vi "PCO_GetCOCRuntime.vi"(8 "error in (no error)":errorcluster {"code" format="%x"}, 11 "ph":u64) -> (0 "error out":errorcluster {"code" format="%x"}, 1 "dwTime_s":u32, 2 "ErrorMessage":i32 format="%x", 3 "ph out":u64, 5 "dwTime_ns":u32)   [LabVIEW 2020, in "SDK.lvlib" / "TimingControl.lvlib"]
doc: "<b>Description:</b>\nThis function can be used to calculate the current frame rate of the camera.\nThe returned values describe exactly how much time is required to take a single image. The resulting time is calculated inside the camera and depends on the settings of the timing and sensor parameters. To cover the full range of possible times it is splitted in two parts. Parameter dwTime_s gives the number of seconds and dwTime_ns gives the number of nano seconds in the range from 0 to 999999999 ns.\nIf external exposure is active, the returned value does describe the readout time only.\n\n<b>Supported camera type:</b>\nAll cameras\n\n<b>Descriptor dependency:</b>\nNone"
uses:
  TimingControl.lvlib
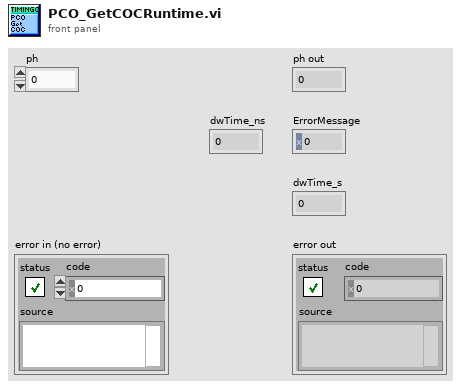
[diagram p1: front panel]
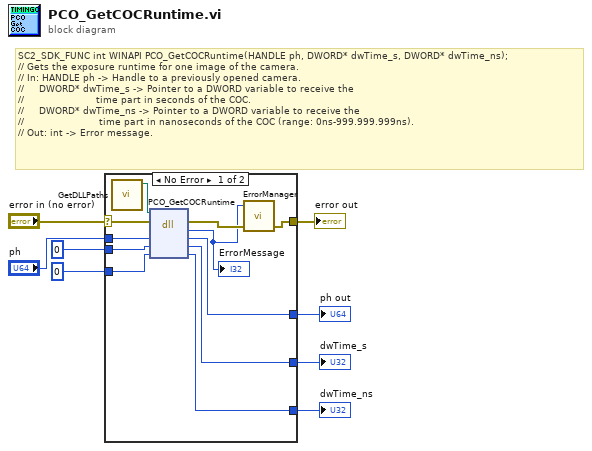
[diagram p0: block diagram]
diagram:
  # "SC2_SDK_FUNC int WINAPI PCO_GetCOCRuntime(HANDLE ph, DWORD* dwTime_s, DWORD* dwTime_ns);\n// Gets the exposure runtime for one image of the camera.\n// In: HANDLE ph -> Handle to a previously opened camera.\n//     DWORD* dwTime_s -> Pointer to a DWORD variable to receive the\n//                        time part in seconds of the COC.\n//     DWORD* dwTime_ns -> Pointer to a DWORD variable to receive the\n//                         time part in nanoseconds of the COC (range: 0ns-999.999.999ns).\n// Out: int -> Error message."
  n1 = case shown="No Error" "error in (no error)" {
    selector: "error in (no error)" -> [w13 w23]
    tunnel: "ph" -> [w19 w22]
    tunnel: [w18 w22] -> w7
    tunnel: u32 0 ("dwTime_s") -> [w17 w21]
    tunnel: [w16 w21] -> w5
    tunnel: u32 0 ("dwTime_ns") -> [w15 w20]
    tunnel: [w14 w20] -> w3
    tunnel: [w11 w23] -> w2
    frame No Error {
      n2 = call "GetDLLPaths.vi"() -> ("SC2_Cam_Path"=w9:path)  [unwired: 9 in, 2 out]
      n3 = dll-call lib="?" fn="PCO_GetCOCRuntime"(path in=w9, error in=w13, "ph"=w19, "dwTime_s"=w17, "dwTime_ns"=w15) -> (error out=w12:errorcluster, "return type"=w10:i32, "ph"=w18:u64, "dwTime_s"=w16:u32, "dwTime_ns"=w14:u32)  [unwired: 1 in, 1 out]
      "ErrorMessage" <- w10
      n4 = call "ErrorManager.vi"("error in (no error)"=w12, "error code"=w10) -> ("error out"=w11:errorcluster)  [unwired: 3 in]
    }
    frame Error {
    }
  }
  "ph out" <- w7
  "dwTime_s" <- w5
  "dwTime_ns" <- w3
  "error out" <- w2
